vi "Poly Read Config API.vi"   [LabVIEW 2021, in "Configuration.lvlib"]
uses:
  Imposible_Snake_v2/LVApp/Architecture/Modules/Configuration/Configuration.lvlib
  Imposible_Snake_v2/LVApp/Modules/Sound Manager/Sound Manager.lvlib
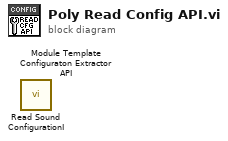
[diagram p0: block diagram]
diagram:
  n1 = call "Read Sound ConfigurationI.vi"() -> ()  [unwired: 10 in, 2 out]
  n2 = call "Module Template Configuraton Extractor API.vi"() -> ()  [unwired: 10 in, 2 out]
